vi "Truncate Kernel.vi"(9 "Array Element Parameters":T1, 11 "Kernel in":sgl[][](array[numeric])) -> (3 "Kernel out":sgl[][](array[numeric]))   [LabVIEW 2021, in "Arrays.lvlib"]
uses:
  Arrays.lvlib
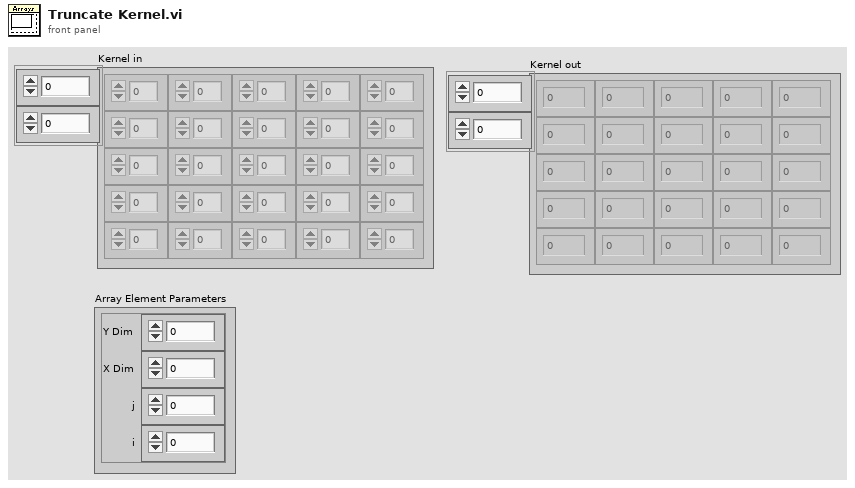
[diagram p1: front panel]
types:
  T1 = cluster{"Y Dim":i32, "X Dim":i32, "j":i32, "i":i32}
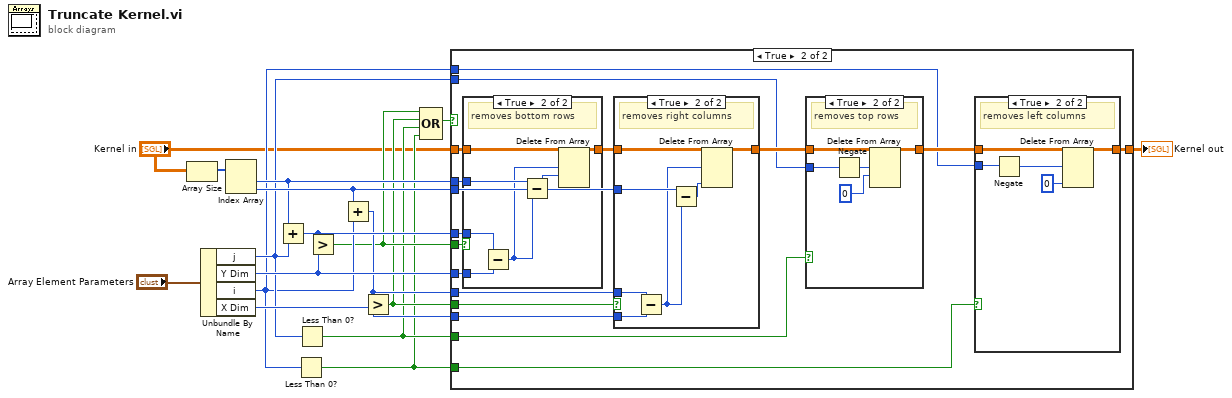
[diagram p0: block diagram]
diagram:
  n1 = Array Size(array="Kernel in") -> (size(s)=w16:i32[])
  n2 = Unbundle By Name("Array Element Parameters") -> ("j"=w9:i32, "Y Dim"=w15:i32, "i"=w8:i32, "X Dim"=w12:i32)
  n3 = Index Array(array=w16) -> (element #1=w10:i32, element #2=w11:i32)  [unwired: 2 in]
  n4 = Add(x=w10, y=w9) -> (x+y=w14:i32)
  n5 = Less Than 0?(x=w8) -> (x < 0?=w4:bool)
  n6 = Less Than 0?(x=w9) -> (x < 0?=w5:bool)
  n7 = Greater?(x=w14, y=w15) -> (0:w7:bool)
  n8 = Add(x=w11, y=w8) -> (x+y=w13:i32)
  n9 = Greater?(x=w13, y=w12) -> (0:w6:bool)
  n10 = Compound Arithmetic op=OR(w7, w6, w5, w4) -> (w3:bool)
  n11 = case shown="True" w3 {
    tunnel: "Kernel in" -> [w18 w35]
    tunnel: w15 -> [_ w34]
    tunnel: w14 -> [_ w33]
    tunnel: w13 -> [_ w31]
    tunnel: w12 -> [_ w30]
    tunnel: w11 -> [_ w29]
    tunnel: w10 -> [_ w27]
    tunnel: [w18 w25] -> w2
    tunnel: w9 -> [_ w24]
    tunnel: w8 -> [_ w23]
    tunnel: w7 -> [_ w22]
    tunnel: w6 -> [_ w21]
    tunnel: w5 -> [_ w20]
    tunnel: w4 -> [_ w19]
    frame False {
    }
    frame True {
      n12 = case shown="True" w22 {
        tunnel: w35 -> [w56 w63]
        tunnel: w34 -> [_ w60]
        tunnel: w33 -> [_ w61]
        tunnel: [w56 w62] -> w32
        tunnel: w27 -> [_ w59]
        frame False {
        }
        frame True {
          # "removes bottom rows"
          n13 = Subtract(x=w61, y=w60) -> (x-y=w58:i32)
          n14 = Subtract(x=w59, y=w58) -> (x-y=w57:i32)
          n15 = Delete From Array(array=w63, length=w58, index (row)=w57) -> (array with subset deleted=w62:sgl[][])  [unwired: 1 in, 1 out]
        }
      }
      n16 = case shown="True" w21 {
        tunnel: w32 -> [w48 w55]
        tunnel: w30 -> [_ w52]
        tunnel: w31 -> [_ w53]
        tunnel: [w48 w54] -> w28
        tunnel: w29 -> [_ w51]
        frame False {
        }
        frame True {
          # "removes right columns"
          n17 = Subtract(x=w53, y=w52) -> (x-y=w50:i32)
          n18 = Subtract(x=w51, y=w50) -> (x-y=w49:i32)
          n19 = Delete From Array(array=w55, length=w50, index (col)=w49) -> (array with subset deleted=w54:sgl[][])  [unwired: 1 in, 1 out]
        }
      }
      n20 = case shown="True" w20 {
        tunnel: w28 -> [w42 w47]
        tunnel: [w42 w46] -> w26
        tunnel: w24 -> [_ w45]
        frame False {
        }
        frame True {
          # "removes top rows"
          n21 = Negate(x=w45) -> (-x=w44:i32)
          n22 = Delete From Array(array=w47, length=w44, index (row)=0) -> (array with subset deleted=w46:sgl[][])  [unwired: 1 in, 1 out]
        }
      }
      n23 = case shown="True" w19 {
        tunnel: w26 -> [w36 w41]
        tunnel: [w36 w40] -> w25
        tunnel: w23 -> [_ w39]
        frame False {
        }
        frame True {
          # "removes left columns"
          n24 = Negate(x=w39) -> (-x=w38:i32)
          n25 = Delete From Array(array=w41, length=w38, index (col)=0 ("disabled index (col)")) -> (array with subset deleted=w40:sgl[][])  [unwired: 1 in, 1 out]
        }
      }
    }
  }
  "Kernel out" <- w2
